vi "TouchMux Sub.vi"(5 "Watch for T3 Pressed":bool, 6 "Watch for T2 Pressed":bool, 7 "Watch for T1 Pressed":bool, 8 "And-Operation":bool, 9 "Connection":T1) -> (0 "t3":bool, 1 "t2":bool, 2 "t1":bool, 3 "Result Value":i16, 4 "watch-result":bool)   [LabVIEW 2010]
uses:
  mindsensors-library.llb/PadSelectorInput.ctl
  mindsensors-library.llb/MerlotRadioButton.ctl
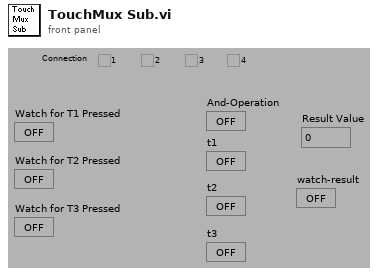
[diagram p1: front panel]
types:
  T1 = typedef "PadSelectorInput.ctl" = enum32{"0", "1", "2", "3", "4"}
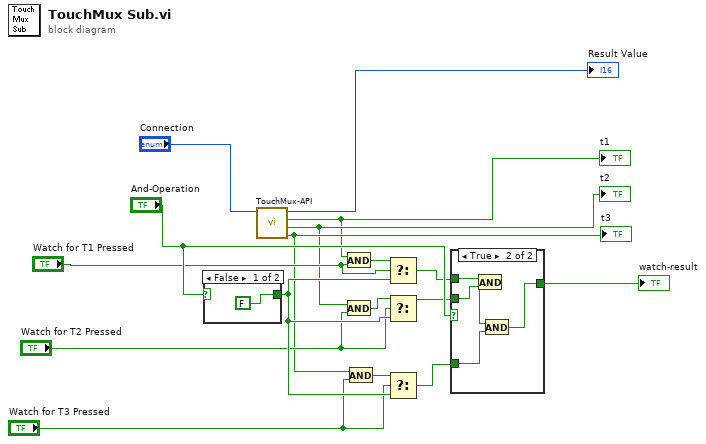
[diagram p0: block diagram]
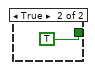
[diagram p2: hidden frame]
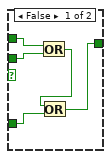
[diagram p3: hidden frame]
diagram:
  n1 = case shown="False" "And-Operation" {
    tunnel: [FALSE ("f") TRUE ("f")] -> w16
    frame False {
    }
    frame True {
    }
  }
  n2 = call "TouchMux-API.vi"("Connection"="Connection") -> ("t3"=w5:bool, "t2"=w4:bool, "t1"=w3:bool, "Result Value"=→"Result Value":i16)  [unwired: 7 in]
  "t3" <- w5
  "t2" <- w4
  "t1" <- w3
  n3 = And(x=w3, y="Watch for T1 Pressed") -> (x .and. y?=w8:bool)
  n4 = And(x=w4, y="Watch for T2 Pressed") -> (x .and. y?=w11:bool)
  n5 = And(x=w5, y="Watch for T3 Pressed") -> (x .and. y?=w14:bool)
  n6 = Select(t=w8, s="Watch for T1 Pressed", f=w16) -> (s? t:f=w7:bool)
  n7 = Select(t=w11, s="Watch for T2 Pressed", f=w16) -> (s? t:f=w10:bool)
  n8 = Select(t=w14, s="Watch for T3 Pressed", f=w16) -> (s? t:f=w13:bool)
  n9 = case shown="True" "And-Operation" {
    tunnel: [w20 w28] -> w6
    tunnel: w7 -> [w24 w27]
    tunnel: w10 -> [w23 w26]
    tunnel: w13 -> [w21 w25]
    frame False {
      n10 = Or(x=w24, y=w23) -> (x .or. y?=w22:bool)
      n11 = Or(x=w22, y=w21) -> (x .or. y?=w20:bool)
    }
    frame True {
      n12 = And(x=w27, y=w26) -> (x .and. y?=w29:bool)
      n13 = And(x=w29, y=w25) -> (x .and. y?=w28:bool)
    }
  }
  "watch-result" <- w6
